vi "Set Date and Time.vi"(8 "error in (no error)":errorcluster, 10 "Data and Time":timestamp, 11 "VISA resource name":refnum<visa-resource-name>) -> (0 "error out":errorcluster, 3 "VISA resource name out":refnum<visa-resource-name>)   [LabVIEW 2014, in "Fluke 190 Series II.lvlib"]
doc: "Sets the real time date and time."
uses:
  Fluke 190 Series II.lvlib
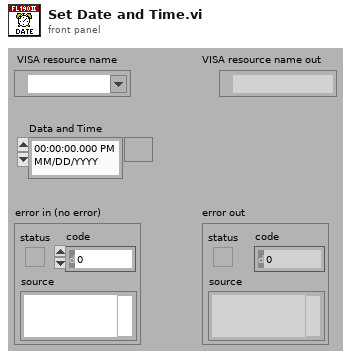
[diagram p1: front panel]
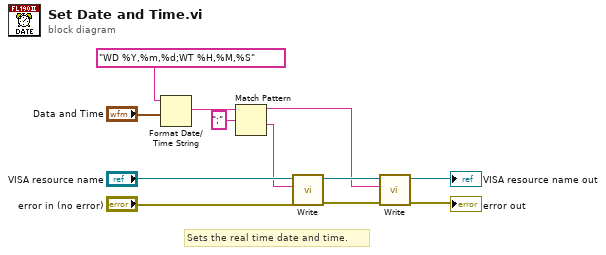
[diagram p0: block diagram]
diagram:
  # "Sets the real time date and time."
  n1 = Format Date/Time String(time format string (%c)="WD %Y,%m,%d;WT %H,%M,%S", seconds (now)="Data and Time") -> (date/time string=w4:string)  [unwired: 1 out]
  n2 = Match Pattern(string=w4, regular expression=";") -> (before substring=w1:string, after substring=w2:string)  [unwired: 3 out]
  n3 = call "Write.vi"("error in (no error)"="error in (no error)", "Write Buffer"=w2, "VISA resource name"="VISA resource name") -> ("error out"=w9:errorcluster, "VISA resource name out"=w10:refnum<visa-resource-name>)  [unwired: 7 out]
  n4 = call "Write.vi"("error in (no error)"=w9, "Write Buffer"=w1, "VISA resource name"=w10) -> ("error out"=→"error out":errorcluster, "VISA resource name out"=→"VISA resource name out":refnum<visa-resource-name>)  [unwired: 7 out]
